vi "SetRGB.vi"(0 "ColorRGB in":refnum<class "ColorRGB.lvclass">, 5 "R":u8, 7 "G":u8, 9 "B":u8, 11 "error in (no error)":errorcluster) -> (4 "ColorRGB out":refnum<class "ColorRGB.lvclass">, 15 "error out":errorcluster)   [LabVIEW 2021, in "Picture2D.lvlib" / "ColorRGB.lvclass"]
uses:
  ColorRGB.lvclass
  C:/GitHub/Picture2D/src/Color/Color.lvclass
  ColorRGB.lvclass/ColorRGB.ctl
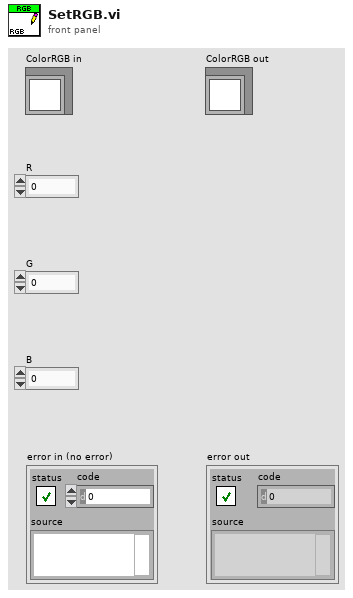
[diagram p1: front panel]
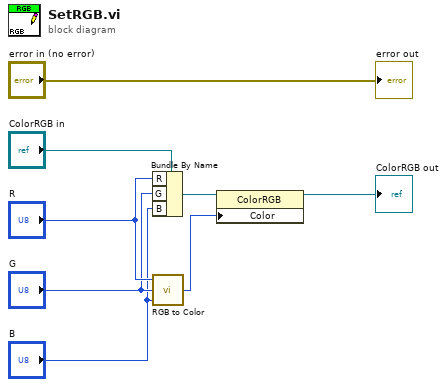
[diagram p0: block diagram]
diagram:
  n1 = Bundle By Name(cluster="ColorRGB in", "R"="R", "G"="G", "B"="B") -> (w2:refnum<class "ColorRGB.lvclass">)
  n2 = call <vilib>:"RGB to Color.vi"("B"="B", "G"="G", "R"="R") -> ("Color"=w1:u32)
  n3 = property class="ColorRGB"(reference=w2, "Color"=w1) -> (reference out=→"ColorRGB out":refnum<class "ColorRGB.lvclass">)  [unwired: 1 in, 1 out]
  "error out" <- "error in (no error)"
